vi "grabber control buttons.vi"() -> ()   [LabVIEW 2012]
panel:
  in  "grabber control buttons":T1
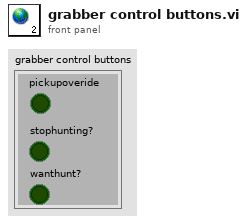
[diagram p1: front panel]
types:
  T1 = cluster{"pickupoveride":bool, "stophunting?":bool, "wanthunt?":bool}
diagram:
